vi "closeLog.vi"(8 "error in (no error)":errorcluster, 11 "Logger in":refnum<class "Log.lvclass">) -> (0 "error out":errorcluster, 3 "Logger out":refnum<class "Log.lvclass">)   [LabVIEW 2013, in "Log.lvlib" / "Log.lvclass"]
uses:
  <userlib>/Common/Log/Log/Log.lvclass
  <userlib>/Common/Log/Log/Log.lvclass/Log.ctl
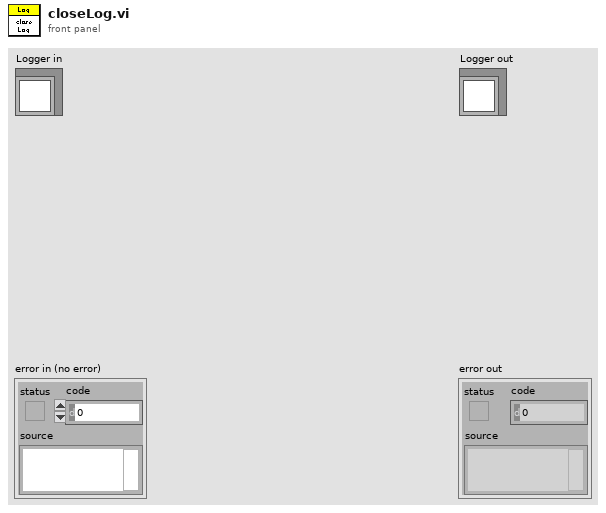
[diagram p1: front panel]
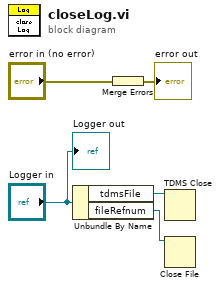
[diagram p0: block diagram]
diagram:
  n1 = Unbundle By Name("Logger in") -> ("tdmsFile"=w2:refnum<k34>, "fileRefnum"=w1:refnum<file>)
  n2 = Merge Errors("error in (no error)") -> (→"error out":errorcluster)
  n3 = TDMS Close(11:w2) -> ()  [unwired: 1 in, 2 out]
  n4 = Close File(refnum=w1) -> ()  [unwired: 1 in, 2 out]
  "Logger out" <- "Logger in"
